vi "ryTimer Close.vi"(8 "error in (no error)":errorcluster, 11 "Timer in":refnum<class "ryTimer.lvclass">) -> (0 "error out":errorcluster)   [LabVIEW 2021, in "ryTimer.lvclass"]
doc: "Releases and destroys the timer."
uses:
  ryTimer.lvclass
  ryTimer.lvclass/ryTimer.ctl
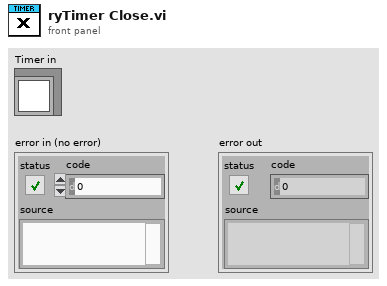
[diagram p1: front panel]
types:
  T1 = typedef "ryTimer.lvclass/ryTimer Properties.ctl" = cluster{"Wait Time (ms)":u32, "Is Running":bool, "Last Ticks":u32, "Emit":refnum<queue>}
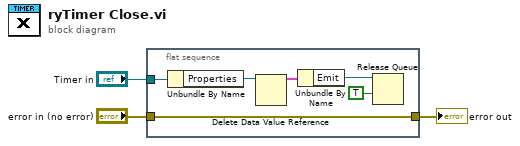
[diagram p0: block diagram]
diagram:
  n1 = flat-sequence {
    tunnel: "Timer in" -> [w6]
    tunnel: [w7] -> w2
    tunnel: "error in (no error)" -> [w7]
    frame #0 {
      n2 = Unbundle By Name(w6) -> ("Properties"=w5:refnum<data-value>)
      n3 = Delete Data Value Reference(data value reference=w5) -> (data value=w4:T1)  [unwired: 1 in, 1 out]
      n4 = Unbundle By Name(w4) -> ("Emit"=w8:refnum<queue>)
      n5 = Release Queue(queue=w8, force destroy? (F)=TRUE) -> ()  [unwired: 1 in, 3 out]
    }
  }
  "error out" <- w2
